vi "SingleTank (SubVI).vi"(6 "H0 [cm]":dbl, 7 "C":dbl=32.0, 9 "HLimit [cm]":dbl=40.0, 10 "T0 [s]":dbl=0.01, 11 "q [cm3/s]":dbl=100.0) -> (2 "Q [cm3/s]":dbl, 3 "H [cm]":dbl)   [LabVIEW 2020]
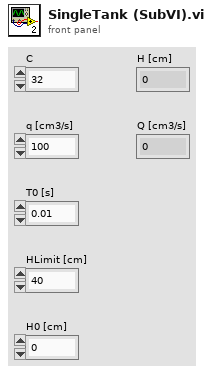
[diagram p1: front panel]
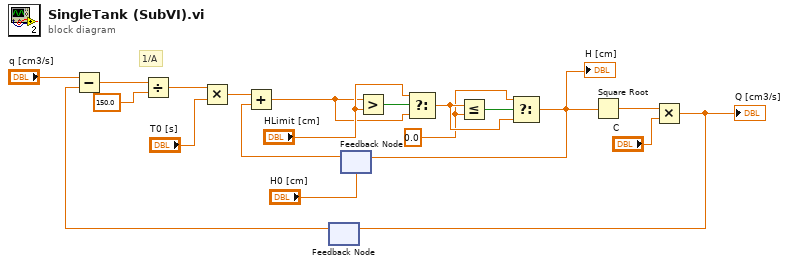
[diagram p0: block diagram]
diagram:
  w16 = 0.0 ("y")
  # "1/A"
  n1 = feedback #1() -> (w10:dbl)  [unwired: 1 in]
  n2 = Subtract(x="q [cm3/s]", y=w10) -> (x-y=w2:dbl)
  n3 = Divide(x=w2, y=150.0) -> (x/y=w9:dbl)
  n4 = Multiply(x=w9, y="T0 [s]") -> (x*y=w4:dbl)
  n5 = feedback #2("H0 [cm]") -> (w5:dbl)
  n6 = Add(x=w4, y=w5) -> (x+y=w13:dbl)
  n7 = Greater?(x=w13, y="HLimit [cm]") -> (0:w12:bool)
  n8 = Select(t="HLimit [cm]", s=w12, f=w13) -> (s? t:f=w17:dbl)
  n9 = Less Or Equal?(x=w17, y=w16) -> (x <= y?=w15:bool)
  n10 = Select(t=w16, s=w15, f=w17) -> (s? t:f=w19:dbl)
  "H [cm]" <- w19
  n11 = feedback-in #2(w19) -> ()
  n12 = Square Root(x=w19) -> (sqrt(x)=w18:dbl)
  n13 = Multiply(x=w18, y="C") -> (x*y=w11:dbl)
  "Q [cm3/s]" <- w11
  n14 = feedback-in #1(w11) -> ()
